vi "Tracker_v2_test_acq_comms.vi"() -> ()   [LabVIEW 2016]
panel:
  in  "Play/Pause":bool
  in  "Stop Button":bool
  out "Read buffer":string
  out "Timestamp":timestamp
  in  "VISA resource name in":refnum<visa-resource-name>="ASRL3::INSTR"
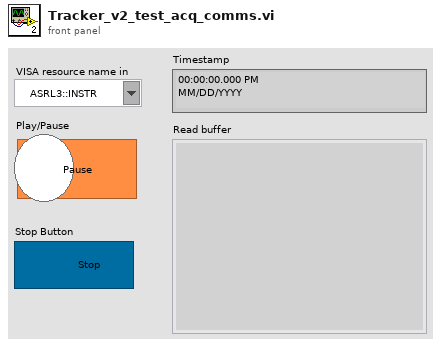
[diagram p1: front panel]
types:
  T1 = cluster{"Data acquisition status":refnum<notifier>, "Play/Pause status":refnum<notifier>, "Recording status":refnum<notifier>}
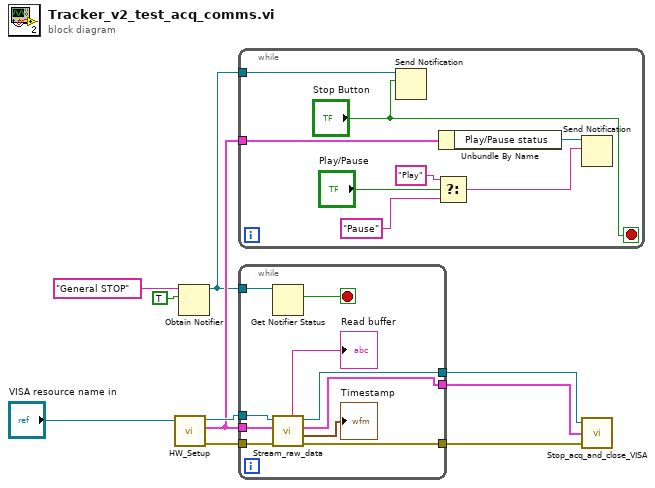
[diagram p0: block diagram]
diagram:
  n1 = call "HW_Setup.vi"("VISA resource name in"="VISA resource name in") -> ("VISA resource name out"=w9:refnum<visa-resource-name>, "Data flow controls"=w4:T1, "error out"=w8:errorcluster)  [unwired: 2 in, 1 out]
  n2 = Obtain Notifier(name (unnamed)="General STOP", notification data type=TRUE) -> (notifier out=w1:refnum<notifier>)  [unwired: 2 in, 2 out]
  n3 = while {
    tunnel: w4 -> [w18]
    tunnel: w1 -> [w12]
    stop <- "Stop Button" stop-if-true
    n4 = Send Notification(notification="Stop Button", notifier=w12) -> ()  [unwired: 1 in, 2 out]
    n5 = Select(t="Play", s="Play/Pause", f="Pause") -> (s? t:f=w15:string)
    n6 = Unbundle By Name(w18) -> ("Play/Pause status"=w17:refnum<notifier>)
    n7 = Send Notification(notification=w15, notifier=w17) -> ()  [unwired: 1 in, 2 out]
  }
  n8 = while {
    tunnel: w9 -> [w28]
    tunnel: [w23] -> w7
    tunnel: w4 -> [w27]
    tunnel: [w22] -> w6
    tunnel: w8 -> [w26]
    tunnel: [w21] -> w5
    tunnel: w1 -> [w20]
    stop <- w19 stop-if-true
    n9 = Get Notifier Status(notifier=w20) -> (current notification=w19:bool)  [unwired: 1 in, 4 out]
    n10 = call "Stream_raw_data.vi"("error in"=w26, "Data flow controls"=w27, "VISA resource name in"=w28) -> ("error out"=w21:errorcluster, "Timestamp"=→"Timestamp":timestamp, "Data flow controls out"=w22:T1, "VISA resource name out"=w23:refnum<visa-resource-name>, "Read buffer"=→"Read buffer":string)  [unwired: 4 in]
  }
  n11 = call "Stop_acq_and_close_VISA.vi"("error in"=w5, "Data flow controls in"=w6, "VISA resource name in"=w7) -> ()  [unwired: 2 out]
